vi "Get Replay Data From File.vi"(7 "V at Max RPM":dbl, 8 "error in (no error)":errorcluster, 10 "Memory Size (number)":i32, 11 "Item Ref in":T1 format="%.0x") -> (0 "error out":errorcluster, 2 "DBL Data":dbl[](array[numeric]), 3 "DAC Data":i16[](array[numeric]))   [LabVIEW 2011, in "Engine Sim System Explorer.lvlib"]
uses:
  Engine Sim System Explorer.lvlib
  <vilib>/NI Veristand/Custom Device API/Custom Device Item Ref.ctl
  TypeDefs/Data Replay Data Selection Method.ctl
  Shared/Engine Simulation Global.vi
  <vilib>/NI Veristand/Custom Device API/Get Item Property (U16).vi
  <vilib>/NI Veristand/Custom Device API/Get Item Property (Double).vi
  <vilib>/NI Veristand/Custom Device API/Get Item Property (Boolean).vi
  <vilib>/NI Veristand/Custom Device API/Get Item Property (String).vi
  <vilib>/NI Veristand/Custom Device API/Get Item Property (U32).vi
  <vilib>/NI Veristand/Custom Device API/Get Item Property (I32).vi
  <vilib>/NI Veristand/Custom Device API/Get Item Property (Dependent File).vi
  <vilib>/NI Veristand/Custom Device API/Custom Device API.lvlib
  Engine Simulation Shared.lvlib
  Data File Loader/Engine Sim File Interface.lvlib
  <userlib>/AES/RT/AES RT.lvlib
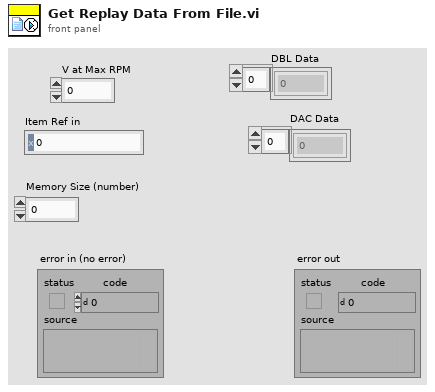
[diagram p1: front panel]
types:
  T1 = typedef "Custom Device API.lvlib/Custom Device Item Ref.ctl" = u64
  T2 = typedef "Engine Sim System Explorer.lvlib/Data Replay Data Selection Method.ctl" = enum32{"Manual", "AutoVRCrank"}
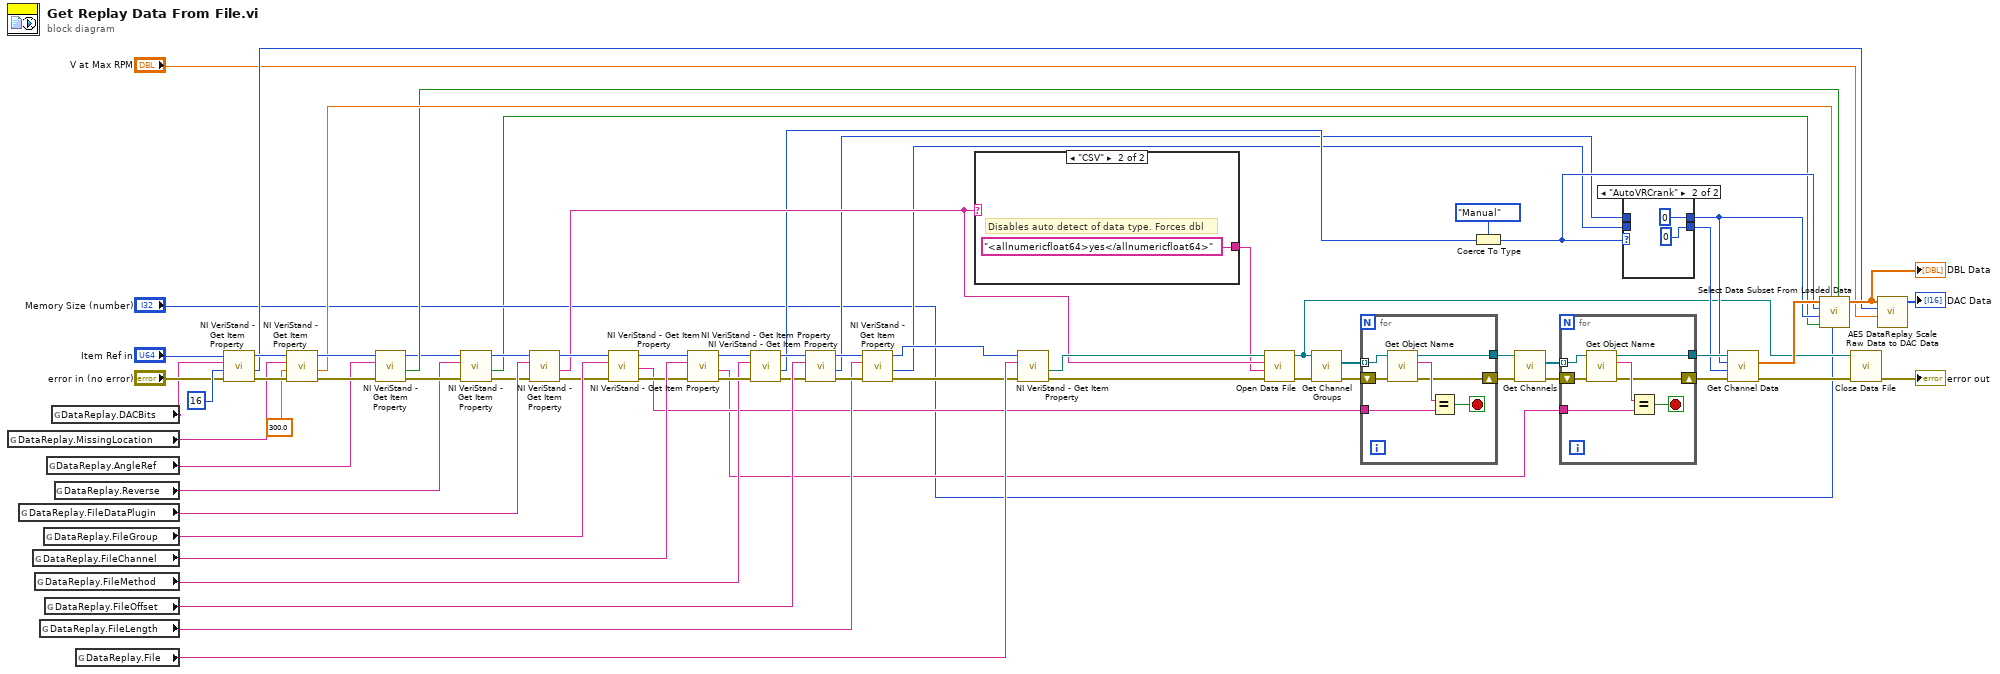
[diagram p0: block diagram]
diagram:
  n1 = global read "Engine Simulation Global.vi" "DataReplay.MissingLocation"() -> (w63:string)
  n2 = global read "Engine Simulation Global.vi" "DataReplay.FileDataPlugin"() -> (w58:string)
  n3 = global read "Engine Simulation Global.vi" "DataReplay.FileChannel"() -> (w52:string)
  n4 = global read "Engine Simulation Global.vi" "DataReplay.FileMethod"() -> (w48:string)
  n5 = global read "Engine Simulation Global.vi" "DataReplay.FileLength"() -> (w42:string)
  n6 = global read "Engine Simulation Global.vi" "DataReplay.FileGroup"() -> (w55:string)
  n7 = global read "Engine Simulation Global.vi" "DataReplay.FileOffset"() -> (w46:string)
  n8 = global read "Engine Simulation Global.vi" "DataReplay.AngleRef"() -> (w59:string)
  n9 = global read "Engine Simulation Global.vi" "DataReplay.DACBits"() -> (w64:string)
  n10 = global read "Engine Simulation Global.vi" "DataReplay.Reverse"() -> (w2:string)
  n11 = global read "Engine Simulation Global.vi" "DataReplay.File"() -> (w40:string)
  n12 = call-poly <vilib>:"NI VeriStand - Get Item Property.vi"("error in (no error)"="error in (no error)", "Default Value"=u16 16, "Property Name"=w64, "Item Ref in"="Item Ref in") -> ("error out"=w67:errorcluster, "Value"=w9:u16, "Item Ref out"=w68:T1)  [unwired: 4 in, 1 out]
  n13 = call-poly <vilib>:"NI VeriStand - Get Item Property.vi"("error in (no error)"=w67, "Default Value"=300.0, "Property Name"=w63, "Item Ref in"=w68) -> ("error out"=w60:errorcluster, "Value"=w20:dbl, "Item Ref out"=w61:T1)  [unwired: 4 in, 1 out]
  n14 = call-poly <vilib>:"NI VeriStand - Get Item Property.vi"("error in (no error)"=w60, "Property Name"=w59, "Item Ref in"=w61) -> ("error out"=w57:errorcluster, "Value"=w19:bool, "Item Ref out"=w4:T1)  [unwired: 5 in, 1 out]
  n15 = call-poly <vilib>:"NI VeriStand - Get Item Property.vi"("error in (no error)"=w57, "Property Name"=w2, "Item Ref in"=w4) -> ("error out"=w5:errorcluster, "Value"=w1:bool, "Item Ref out"=w3:T1)  [unwired: 5 in, 1 out]
  n16 = call-poly <vilib>:"NI VeriStand - Get Item Property.vi"("error in (no error)"=w5, "Property Name"=w58, "Item Ref in"=w3) -> ("error out"=w54:errorcluster, "Value"=w37:string, "Item Ref out"=w56:T1)  [unwired: 5 in, 1 out]
  n17 = call-poly <vilib>:"NI VeriStand - Get Item Property.vi"("error in (no error)"=w54, "Property Name"=w55, "Item Ref in"=w56) -> ("error out"=w51:errorcluster, "Value"=w32:string, "Item Ref out"=w53:T1)  [unwired: 5 in, 1 out]
  n18 = call-poly <vilib>:"NI VeriStand - Get Item Property.vi"("error in (no error)"=w51, "Property Name"=w52, "Item Ref in"=w53) -> ("error out"=w49:errorcluster, "Value"=w27:string, "Item Ref out"=w50:T1)  [unwired: 5 in, 1 out]
  n19 = call-poly <vilib>:"NI VeriStand - Get Item Property.vi"("error in (no error)"=w49, "Property Name"=w48, "Item Ref in"=w50) -> ("error out"=w45:errorcluster, "Value"=w23:u32, "Item Ref out"=w47:T1)  [unwired: 5 in, 1 out]
  n20 = call-poly <vilib>:"NI VeriStand - Get Item Property.vi"("error in (no error)"=w45, "Property Name"=w46, "Item Ref in"=w47) -> ("error out"=w43:errorcluster, "Value"=w15:i32, "Item Ref out"=w44:T1)  [unwired: 5 in, 1 out]
  n21 = call-poly <vilib>:"NI VeriStand - Get Item Property.vi"("error in (no error)"=w43, "Property Name"=w42, "Item Ref in"=w44) -> ("error out"=w7:errorcluster, "Value"=w16:i32, "Item Ref out"=w41:T1)  [unwired: 5 in, 1 out]
  n22 = case shown="\"CSV\"" w37 {
    tunnel: [_ "<allnumericfloat64>yes</allnumericfloat64>"] -> w36
    frame Default {
    }
    frame "CSV" {
      # "Disables auto detect of data type. Forces dbl"
    }
  }
  n23 = call-poly <vilib>:"NI VeriStand - Get Item Property.vi"("error in (no error)"=w7, "Property Name"=w40, "Item Ref in"=w41) -> ("error out"=w38:errorcluster, "Path"=w39:path)  [unwired: 4 in, 3 out]
  n24 = call "Open Data File.vi"("error in (no error)"=w38, "Additional parameters"=w36, "Data Plugin"=w37, "File Path"=w39) -> ("error out"=w35:errorcluster, "File Ref"=w13:refnum<k20>)  [unwired: 6 in]
  n25 = call "Get Channel Groups.vi"("error in (no error)"=w35, "File Ref in"=w13) -> ("error out"=w34:errorcluster, "Channel Groups"=w33:refnum<k20>[])  [unwired: 7 in, 1 out]
  n26 = for {
    shift-right: [w71] -> w31
    shift-left: w34 -> [w77]
    tunnel: w33 -> [w76] mode=indexing
    tunnel: [w73] -> w30
    tunnel: w32 -> [w72]
    stop <- w74 stop-if-true
    n27 = call "Get Object Name.vi"("error in (no error)"=w77, "Storage Object in"=w76) -> ("error out"=w71:errorcluster, "Name"=w75:string, "Storage Object out"=w73:refnum<k20>)  [unwired: 7 in]
    n28 = Equal?(x=w75, y=w72) -> (x = y?=w74:bool)
  }
  n29 = Coerce To Type(0:w23, 1:Data_Replay_Data_Selection_Method."Manual" ("Data Selection Method")) -> (2:w18:T2)
  n30 = call "Get Channels.vi"("error in (no error)"=w31, "Channel Group in"=w30) -> ("error out"=w29:errorcluster, "Channels"=w28:refnum<k20>[])  [unwired: 7 in, 1 out]
  n31 = for {
    shift-right: [w78] -> w26
    shift-left: w29 -> [w84]
    tunnel: w28 -> [w83] mode=indexing
    tunnel: [w80] -> w25
    tunnel: w27 -> [w79]
    stop <- w81 stop-if-true
    n32 = call "Get Object Name.vi"("error in (no error)"=w84, "Storage Object in"=w83) -> ("error out"=w78:errorcluster, "Name"=w82:string, "Storage Object out"=w80:refnum<k20>)  [unwired: 7 in]
    n33 = Equal?(x=w82, y=w79) -> (x = y?=w81:bool)
  }
  n34 = case shown="\"AutoVRCrank\"" w18 {
    tunnel: [w86 0 ("Count (0: Read All)")] -> w24
    tunnel: [w85 0 ("index")] -> w17
    tunnel: w16 -> [w86 _]
    tunnel: w15 -> [w85 _]
    frame "Manual", Default {
    }
    frame "AutoVRCrank" {
    }
  }
  n35 = call "Get Channel Data.vi"("error in"=w26, "Count (0: Read All)"=w24, "index"=w17, "Channel in"=w25) -> ("error out"=w14:errorcluster, "Signal"=w21:dbl[])  [unwired: 5 in, 1 out]
  n36 = call "Select Data Subset From Loaded Data.vi"("CycleAngle?"=w19, "Memory Size as number"="Memory Size (number)", "MissingTeeth"=w20, "ReverseData"=w1, "Offset"=w17, "Data Selection Method"=w18, "Signal"=w21) -> ("Resampled Data"=w12:dbl[])  [unwired: 2 in, 2 out]
  "DBL Data" <- w12
  n37 = call "Close Data File.vi"("error in (no error)"=w14, "File Ref"=w13) -> ("error out"=→"error out":errorcluster)  [unwired: 9 in]
  n38 = call <userlib>:"AES DataReplay Scale Raw Data to DAC Data.vi"("votlage at max RPM"="V at Max RPM", "DAC bit resolution (16)"=w9, "replay data"=w12) -> ("DAC data"=→"DAC Data":i16[])  [unwired: 8 in]
